vi "SMT_Cell Transfer.vi"(6 "OperatorName":string, 7 "DestinationCellID":string, 8 "error in (no error)":errorcluster caption="错误输入（无错误）", 9 "OriginalCellID":string, 10 "LoadID":string, 11 "Traceability 引用句柄":refnum<k24>) -> (0 "error out":errorcluster caption="错误输出", 2 "SMT_CellTransfer":string, 3 "Traceability 引用句柄输出":refnum<k24>)   [LabVIEW 2014, in "Traceability.lvlib"]
uses:
  D:/webservice/Traceability.dll
  Traceability.dll
  Traceability.lvlib
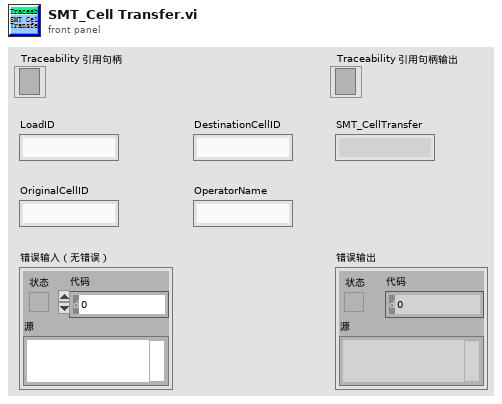
[diagram p1: front panel]
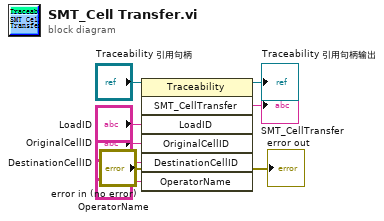
[diagram p0: block diagram]
diagram:
  n1 = invoke class="Traceability" method="SMT_CellTransfer"(reference="Traceability 引用句柄", error in="error in (no error)", "LoadID"="LoadID", "OriginalCellID"="OriginalCellID", "DestinationCellID"="DestinationCellID", "OperatorName"="OperatorName") -> (reference out=→"Traceability 引用句柄输出":refnum<k24>, error out=→"error out":errorcluster, "SMT_CellTransfer"=→"SMT_CellTransfer":string)  [unwired: 1 in, 4 out]
